vi "SRV_PM_Read Packet outside of Receive State Machine.vi"(0 "SRV":refnum<k5>, 11 "error in (no error)":errorcluster) -> (4 "SRV out":refnum<k5>, 6 "Packet Data Field String":string, 8 "Packet":T1 {"Packet Data" format="%.0x"}, 10 "Packet Complete?":bool, 15 "error out":errorcluster)   [LabVIEW 2014]
uses:
  SRV_PM_Packet.ctl
  TCP_Communication/SRV_TCP Settings.ctl
  TCP_Communication/SRV_Package Methods.ctl
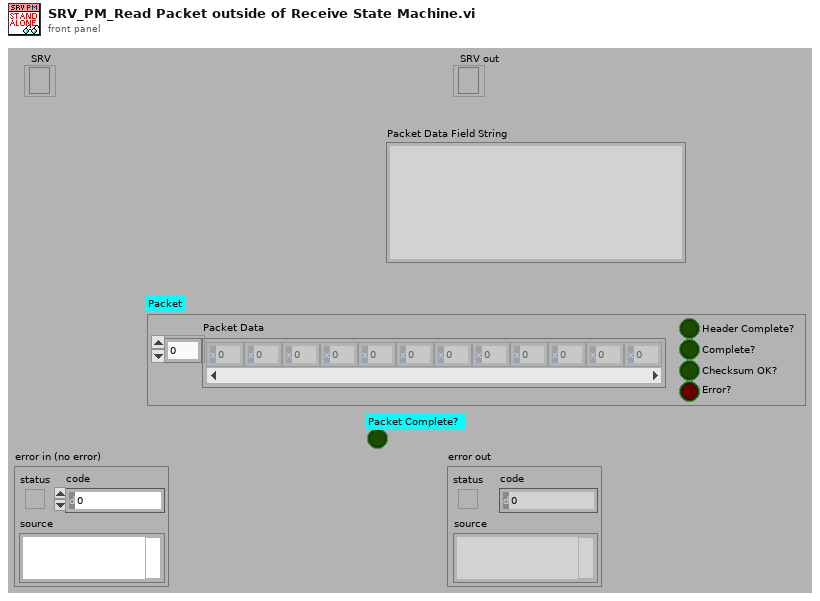
[diagram p1: front panel]
types:
  T1 = typedef "SRV_PM_Packet.ctl" = cluster{"Packet Data":u8[], "Header Complete?":bool, "Complete?":bool, "Checksum OK?":bool, "Error?":bool}
  T2 = typedef "SRV_TCP Settings.ctl" = cluster{"Method":T3, "bytes to read":i32, "timeout ms (1000)":i32}
  T3 = typedef "SRV_Package Methods.ctl" = enum16{"General", "Standard", "CRLF", "Image", "HTML"}
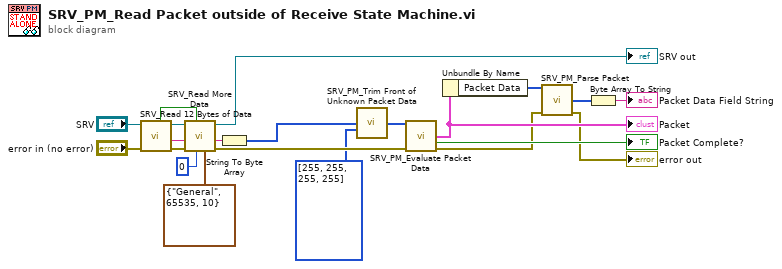
[diagram p0: block diagram]
diagram:
  n1 = call "SRV_Read 12 Bytes of Data.vi"("error in (no error)"="error in (no error)", "SRV In"="SRV") -> ("error out"=w19:errorcluster, "Data out"=w20:string, "SRV Out"=w18:refnum<k5>, "Read more data"=w17:bool)  [unwired: 6 in]
  n2 = call "SRV_Read More Data.vi"("TCP Settings"=T2 {"Method"=enum."General", "bytes to read"=65535, "timeout ms (1000)"=10}, "Delay Before Read (10ms)"=u32 0, "Read More Data? (T)"=w17, "error in (no error)"=w19, "Data in"=w20, "Connection ID"=w18) -> ("error out"=w14:errorcluster, "Data out"=w21:string, "Connection ID out"=→"SRV out":refnum<k5>)  [unwired: 3 in]
  n3 = String To Byte Array(string=w21) -> (unsigned byte array=w12:u8[])
  n4 = call "SRV_PM_Trim Front of Unknown Packet Data.vi"("1D Array"=w12, "Search"=u8[] [255, 255, 255, 255]) -> ("Trimmed 1D Array"=w15:u8[])  [unwired: 12 in, 1 out]
  n5 = call "SRV_PM_Evaluate Packet Data.vi"("Packet Data"=w15, "error in (no error)"=w14) -> ("Packet"=w10:T1, "Packet Complete?"=→"Packet Complete?":bool, "error out"=w5:errorcluster)  [unwired: 9 in, 2 out]
  "Packet" <- w10
  n6 = Unbundle By Name(w10) -> ("Packet Data"=w6:u8[])
  n7 = call "SRV_PM_Parse Packet.vi"("Packet"=w6, "error in (no error)"=w5) -> ("Data Field"=w3:u8[], "error out"=→"error out":errorcluster)  [unwired: 4 in, 8 out]
  n8 = Byte Array To String(unsigned byte array=w3) -> (string=→"Packet Data Field String":string)
